vi "Analyze Image.vi"(11 "path":path) -> (0 "Log Sums":dbl[](array[numeric]), 1 "2D FFT":dbl[][](array[numeric]), 2 "image data":T1, 3 "path out":path)   [LabVIEW 2020]
uses:
  <vilib>/picture/picture.llb/imagedata.ctl
  <vilib>/Analysis/2dsp.llb/2D Real FFT.vi
  <vilib>/Analysis/NI_AALPro.lvlib
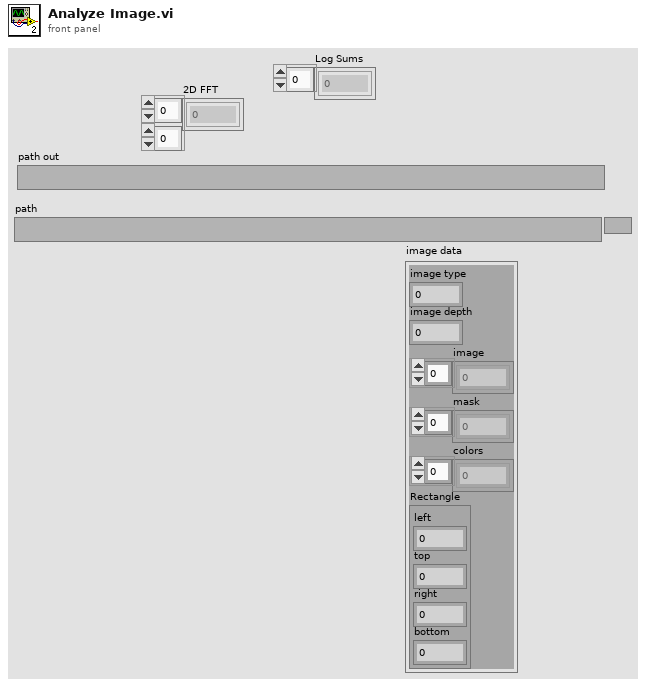
[diagram p1: front panel]
types:
  T1 = typedef "imagedata.ctl" = cluster{"image type":i32, "image depth":i32, "image":u8[], "mask":u8[], "colors":u32[], "Rectangle":cluster{"left":i16, "top":i16, "right":i16, "bottom":i16}}
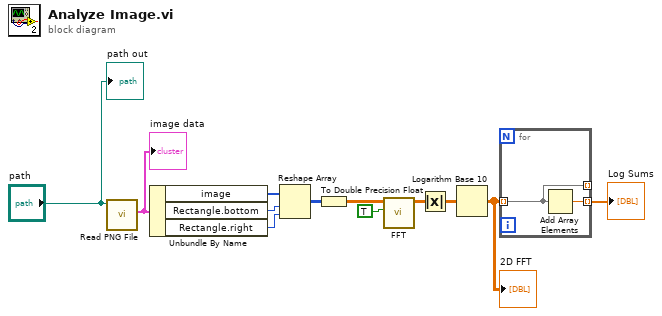
[diagram p0: block diagram]
diagram:
  n1 = call <vilib>:"Read PNG File.vi"("path to PNG file"="path") -> ("image data"=w1:T1)  [unwired: 8 in, 2 out]
  "image data" <- w1
  n2 = Unbundle By Name(w1) -> ("image"=w5:u8[], "Rectangle.bottom"=w6:i16, "Rectangle.right"=w7:i16)
  n3 = Reshape Array(w5, w6, w7) -> (w8:u8[][])
  n4 = To Double Precision Float(number=w8) -> (double precision float=w10:dbl[][])
  n5 = call-poly <vilib>:"FFT.vi"("shift?"=TRUE, "X"=w10) -> ("FFT {X}"=w9:cdb[][])  [unwired: 8 in, 1 out]
  n6 = Absolute Value(x=w9) -> (abs(x)=w12:dbl[][])
  n7 = Logarithm Base 10(1:w12) -> (0:w3:dbl[][])
  "2D FFT" <- w3
  n8 = for {
    tunnel: [w13] -> _ mode=indexing
    tunnel: [w14] -> w2 mode=indexing
    tunnel: w3 -> [w13] mode=indexing
    n9 = Add Array Elements(numeric array=w13) -> (sum=w14:dbl)
  }
  "Log Sums" <- w2
  "path out" <- "path"
